vi "Get_KPRO_data_from_file 2016.vi"(11 "Output File KPRO Test":path=path "c:/KPRO_001.txt") -> (0 "Last_height_of_box":dbl format="%.2f", 1 "Last_depth_to_water":dbl format="%.2f", 2 "Last_depth":dbl format="%.2f", 3 "Output_array":sgl[][](array[numeric]) format="%.2f")   [LabVIEW 2016]
uses:
  controls/KPro Header Control 1.ctl
  <vilib>/Utility/file.llb/Read Delimited Spreadsheet (string).vi
  <vilib>/Utility/file.llb/Read Delimited Spreadsheet (DBL).vi
panel:
  in  "KPRO session report header":T1=["Time(msecs)", "Uncorrected Depth", "Corrected Depth", "Drive_Rate", "Flow", "Feet_of Stainless", "Up Hole Pressure", "IK", "Corrected Pressure", "Atm Pressure", "Depth to water", "Height of box", "Res_Pressure", "Secs_since_1_JAN_1904", "Depth jumps more than 1_foot", "Down hole Pressure"]
  out "first row":string[](array[string])
  out "report_header_length":i32
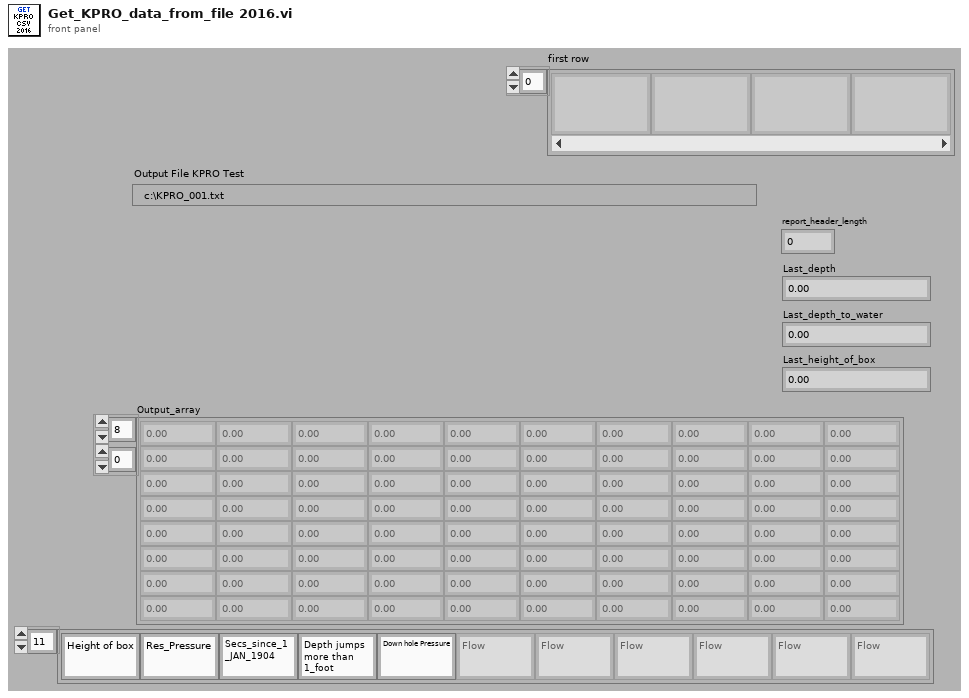
[diagram p1: front panel]
types:
  T1 = typedef "KPro Header Control 1.ctl" = string[]
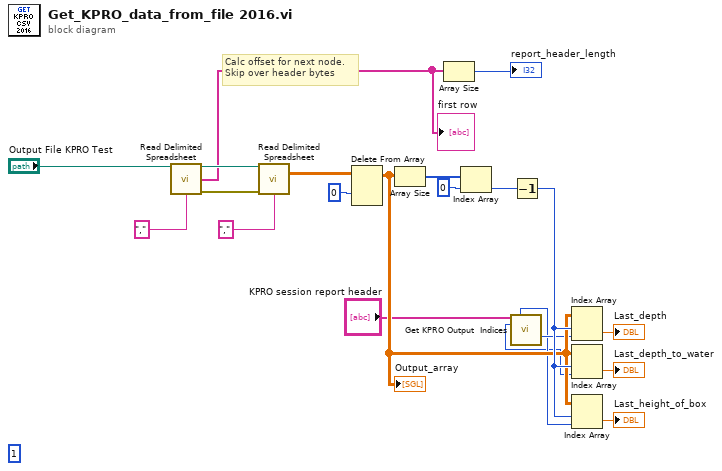
[diagram p0: block diagram]
diagram:
  (unwired) 1 ("number of lines (all:-1)")
  # "Calc offset for next node.\nSkip over header bytes"
  n1 = call-poly <vilib>:"Read Delimited Spreadsheet.vi"("file path (dialog if empty)"="Output File KPRO Test", "delimiter (\\t)"="," ("delimiter (\\t)")) -> ("new file path (Not A Path if cancelled)"=w12:path, "first row"=w11:string[], "error out"=w5:errorcluster)  [unwired: 8 in, 3 out]
  "first row" <- w11
  n2 = call-poly <vilib>:"Read Delimited Spreadsheet.vi"("file path (dialog if empty)"=w12, "error in (no error)"=w5, "delimiter (\\t)"="," ("delimiter (\\t)")) -> ("all rows"=w9:dbl[][])  [unwired: 7 in, 5 out]
  n3 = Delete From Array(array=w9, index (row)=0) -> (array with subset deleted=w8:dbl[][])  [unwired: 2 in, 1 out]
  "Output_array" <- w8
  n4 = Array Size(array=w8) -> (size(s)=w20:i32[])
  n5 = Array Size(array=w11) -> (size(s)=→"report_header_length":i32)
  n6 = Index Array(array=w20, index=0) -> (element=w18:i32)
  n7 = call "Get KPRO Output  Indices.vi"("KPRO Culmulative \ntest report header 2"="KPRO session report header") -> ("Height of Box (global)"=w2:i32, "Depth to Water Table (global)"=w1:i32, "Corrected Depth Index"=w3:i32)  [unwired: 4 in, 8 out]
  n8 = Decrement(x=w18) -> (x-1=w17:i32)
  n9 = Index Array(array=w8, index (row)=w17, index (col)=w3) -> (element=→"Last_depth":dbl)
  n10 = Index Array(array=w8, index (row)=w17, index (col)=w1) -> (element=→"Last_depth_to_water":dbl)
  n11 = Index Array(array=w8, index (row)=w17, index (col)=w2) -> (element=→"Last_height_of_box":dbl)
